vi "cRIO Module Info.vi"(8 "error in":errorcluster, 10 "Module":u16, 11 "Refnum in":refnum<k20>) -> (0 "error out":errorcluster, 2 "cRIO Module Info":T1 {"Serial Number" format="%.0x"; "Vendor and Module ID" format="%.0x"}, 3 "Refnum out":refnum<k20>)   [LabVIEW 2015]
uses:
  <vilib>/rvi/interface/nirviReadWriteControl/nirviReadWriteControl.xnode
  NiFpgaLv.dll
  <vilib>/Utility/error.llb/Error Cluster From Error Code.vi
  <vilib>/rvi/interface/Simulation/niFpgaSimulationCallBeginRW.vi
  <vilib>/rvi/errors/niLvFpgaAdjustHostInterfaceError.vi
  Controls/cRIO Module Info.ctl
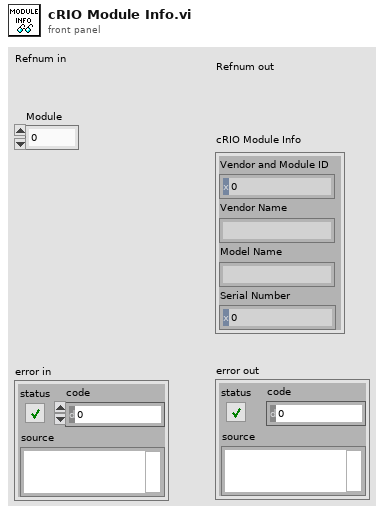
[diagram p1: front panel]
types:
  T1 = typedef "RT Management.lvlib/Module Detection.lvclass/cRIO Module Info.ctl" = cluster{"Vendor and Module ID":u32, "Vendor Name":string, "Model Name":string, "Serial Number":u32}
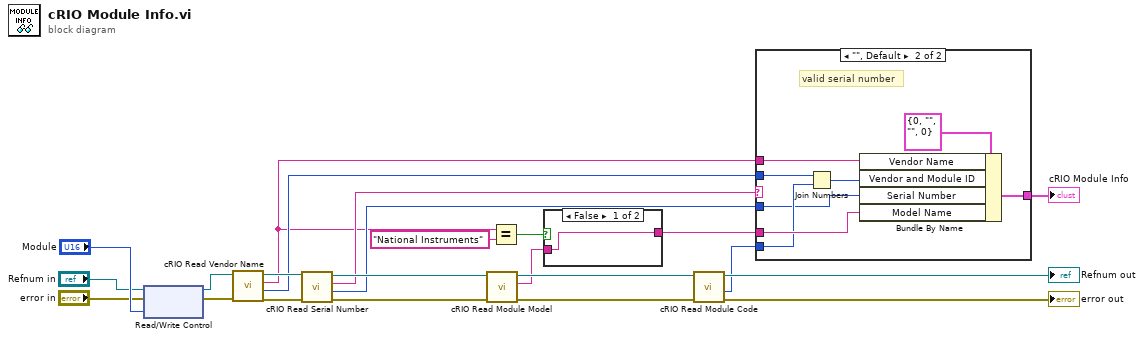
[diagram p0: block diagram]
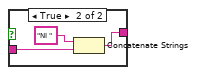
[diagram p2: hidden frame]
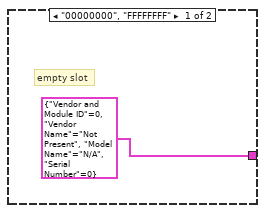
[diagram p3: hidden frame]
diagram:
  n1 = xnode "Read/Write Control"("FPGA VI Reference In"="Refnum in", "error in"="error in", "Module"="Module") -> ("FPGA VI Reference Out"=w17:refnum<k20>, "error out"=w18:errorcluster)
  n2 = call "cRIO Read Vendor Name.vi"("error in"=w18, "Refnum in"=w17) -> ("error out"=w20:errorcluster, "Vendor ID"=w9:u16, "Vendor Name"=w5:string, "Refnum out"=w21:refnum<k20>)  [unwired: 6 in]
  n3 = call "cRIO Read Serial Number.vi"("error in"=w20, "Refnum in"=w21) -> ("error out"=w23:errorcluster, "Serial Number"=w6:u32, "Serial Number String"=w14:string, "Refnum out"=w22:refnum<k20>)  [unwired: 6 in]
  n4 = call "cRIO Read Module Model.vi"("error in"=w23, "Refnum in"=w22) -> ("error out"=w13:errorcluster, "Module Model"=w2:string, "Refnum out"=w12:refnum<k20>)  [unwired: 7 in]
  n5 = Equal?(x=w5, y="National Instruments") -> (x = y?=w3:bool)
  n6 = case shown="False" w3 {
    tunnel: w2 -> [w24 w26]
    tunnel: [w24 w25] -> w1
    frame False {
    }
    frame True {
      n7 = Concatenate Strings("NI " ("string"), w26) -> (w25:string)
    }
  }
  n8 = call "cRIO Read Module Code.vi"("error in"=w13, "Refnum in"=w12) -> ("error out"=→"error out":errorcluster, "Module ID"=w7:u16, "Refnum out"=→"Refnum out":refnum<k20>)  [unwired: 6 in, 1 out]
  n9 = case shown="\"\", Default" w14 {
    tunnel: w5 -> [_ w36]
    tunnel: w1 -> [_ w35]
    tunnel: [T1 {"Vendor and Module ID"=0, "Vendor Name"="Not Present", "Model Name"="N/A", "Serial Number"=0} ("cRIO Module Info") w34] -> w8
    tunnel: w7 -> [_ w33]
    tunnel: w9 -> [_ w32]
    tunnel: w6 -> [_ w31]
    frame "00000000", "FFFFFFFF" {
      # "empty slot"
    }
    frame "", Default {
      # "valid serial number"
      n10 = Join Numbers(hi=w32, lo=w33) -> ((hi.lo)=w29:u32)
      n11 = Bundle By Name(cluster=T1 {"Vendor and Module ID"=0, "Vendor Name"="", "Model Name"="", "Serial Number"=0} ("cRIO Module Info"), "Vendor Name"=w36, "Vendor and Module ID"=w29, "Serial Number"=w31, "Model Name"=w35) -> (w34:T1)
    }
  }
  "cRIO Module Info" <- w8
